vi "Create Read Worker MHLC.vi"(8 "error in (no error)":errorcluster, 10 "Data in":variant, 11 "TCPServer in":refnum<class "DS TCP Server.lvclass">) -> (0 "error out":errorcluster, 3 "TCPServer out":refnum<class "DS TCP Server.lvclass">)   [LabVIEW 2017, in "DS TCP Server.lvlib" / "DS TCP Server.lvclass"]
doc: "Launch a TCP Read Worker to receive incoming data from a Debug Client"
uses:
  DS TCP Server.lvclass
  C:/Program Files (x86)/National Instruments/LabVIEW 2017/vi.lib/addons/_Workers/Library/Classes/Worker/Worker.lvclass
  rql_Create Read Worker.ctl
  <vilib>/addons/_Workers/Library/Classes/Message Queue/Message Queue.lvclass
  Common VIs/DC_UID.ctl
  <vilib>/addons/_Workers/Library/Classes/Message/Priority.ctl
  DS TCP Server.lvclass/DS TCP Server.ctl
  DS TCP Read/Initialization Data.ctl
  DS TCP Read/Response Cases.ctl
  <vilib>/addons/_Workers/Library/Case Label.ctl
  rsp_Connection Notify.ctl
  <vilib>/Utility/error.llb/Error Cluster From Error Code.vi
  <vilib>/ErrorRing/Error Ring.xnode
  DS TCP Read/DS TCP Read.lvclass
  <vilib>/addons/_Workers/Library/Workers.lvlib
  <vilib>/addons/_Workers/Library/Classes/Message/Message.lvclass
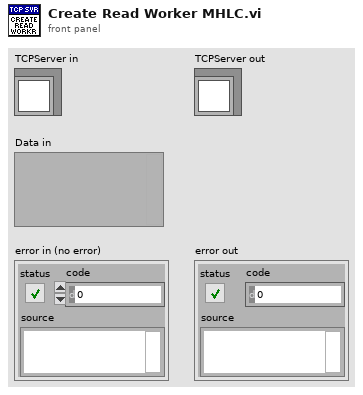
[diagram p1: front panel]
types:
  T1 = typedef "DS TCP Server.lvlib/DS TCP Server.lvclass/rql_Create Read Worker.ctl" = cluster{"Forwarding Q":refnum<class "Message Queue.lvclass">, "DC_UID":T2, "Worker Alias":string, "Message Priority":T3}
  T2 = typedef "DC_UID.ctl" = string
  T3 = typedef "Workers.lvlib/Message.lvclass/Priority.ctl" = enum16{"Low", "Normal", "High"}
  T4 = typedef "DS TCP Server.lvlib/DS TCP Server.lvclass/Connection ID.ctl" = cluster{"Connection Ref":refnum<k5>, "DC_UID":T2, "Message Priority":T3, "IP Address":string}
  T5 = typedef "DS TCP Server.lvlib/DS TCP Server.lvclass/rsp_Connection Notify.ctl" = cluster{"Connected?":bool, "DC_UID":T2, "Message Priority":T3, "IP Address":string}
  T6 = typedef "DS TCP Server.lvlib/DS TCP Read.lvclass/Initialization Data.ctl" = cluster{"Connection ID":refnum<k5>, "Forwarding Queue":refnum<class "Message Queue.lvclass">, "Response Cases":T7}
  T7 = typedef "DS TCP Server.lvlib/DS TCP Read.lvclass/Response Cases.ctl" = cluster{"Connection Lost":T8}
  T8 = typedef "Workers.lvlib/Case Label.ctl" = string
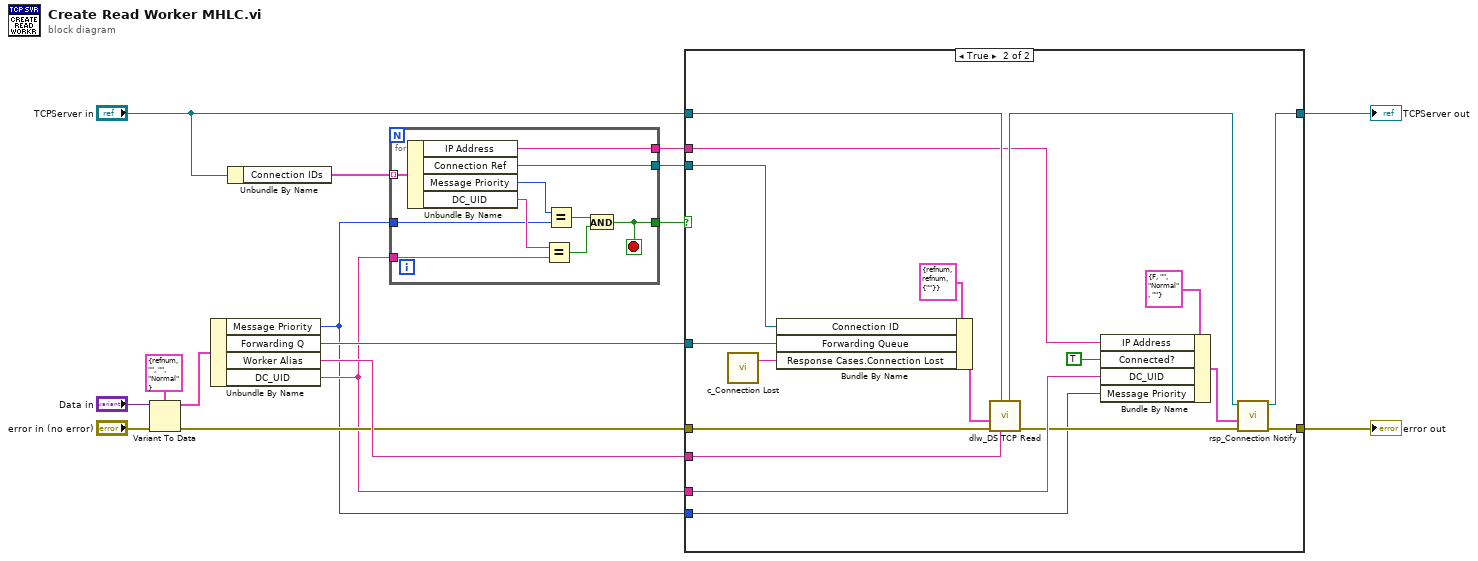
[diagram p0: block diagram]
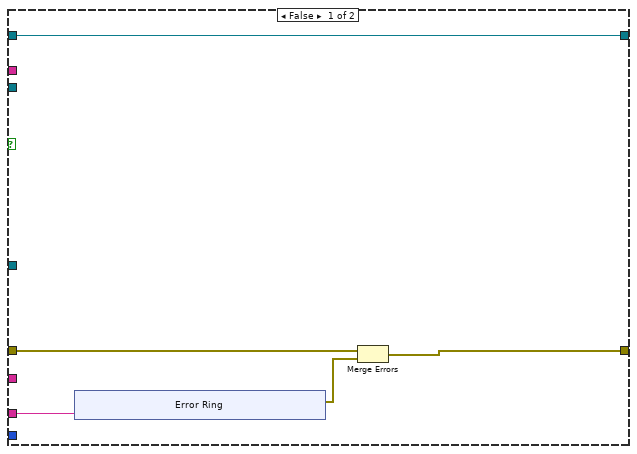
[diagram p2: hidden frame]
diagram:
  n1 = Variant To Data(error in="error in (no error)", type=T1 {"Forwarding Q"=refnum, "DC_UID"="", "Worker Alias"="", "Message Priority"=enum."Normal"} ("Data"), Variant="Data in") -> (data=w10:T1, error out=w7:errorcluster)
  n2 = Unbundle By Name(w10) -> ("Message Priority"=w2:T3, "Forwarding Q"=w11:refnum<class "Message Queue.lvclass">, "Worker Alias"=w12:string, "DC_UID"=w3:T2)
  n3 = Unbundle By Name("TCPServer in") -> ("Connection IDs"=w16:T4[])
  n4 = for {
    tunnel: w16 -> [w26] mode=indexing
    tunnel: w3 -> [w24]
    tunnel: [w18] -> w5
    tunnel: [w23] -> w4
    tunnel: w2 -> [w20]
    tunnel: [w17] -> w1
    stop <- w18 stop-if-true
    n5 = Unbundle By Name(w26) -> ("IP Address"=w17:string, "Connection Ref"=w23:refnum<k5>, "Message Priority"=w21:T3, "DC_UID"=w25:T2)
    n6 = Equal?(x=w25, y=w24) -> (x = y?=w22:bool)
    n7 = Equal?(x=w21, y=w20) -> (x = y?=w19:bool)
    n8 = And(x=w19, y=w22) -> (x .and. y?=w18:bool)
  }
  n9 = case shown="True" w5 {
    tunnel: "TCPServer in" -> [w31 w56]
    tunnel: w3 -> [w28 w55]
    tunnel: [w31 w51] -> w14
    tunnel: [w29 w49] -> w13
    tunnel: w12 -> [_ w48]
    tunnel: w11 -> [_ w46]
    tunnel: w7 -> [w30 w42]
    tunnel: w4 -> [_ w41]
    tunnel: w2 -> [_ w40]
    tunnel: w1 -> [_ w39]
    frame False {
      n10 = xnode "Error Ring"("parameter 0"=w28) -> ("error out"=w27:errorcluster)
      n11 = Merge Errors(w30, w27) -> (w29:errorcluster)
    }
    frame True {
      n12 = call "c_Connection Lost.vi"() -> ("Case Label"=w47:T8)  [unwired: 1 in]
      n13 = Bundle By Name(cluster=T6 {"Connection ID"=refnum, "Forwarding Queue"=refnum, "Response Cases"={"Connection Lost"=""}} ("Initialization Data"), "Connection ID"=w41, "Forwarding Queue"=w46, "Response Cases.Connection Lost"=w47) -> (w45:T6)
      n14 = call "dlw_DS TCP Read.vi"("Worker Alias"=w48, "Caller in"=w56, "error in"=w42, "Initialization Data"=w45) -> ("error out"=w43:errorcluster, "dup Caller out"=w50:refnum<class "DS TCP Server.lvclass">)  [unwired: 5 in, 1 out]
      n15 = Bundle By Name(cluster=T5 {"Connected?"=FALSE, "DC_UID"="", "Message Priority"=enum."Normal", "IP Address"=""} ("Data in"), "IP Address"=w39, "Connected?"=TRUE, "DC_UID"=w55, "Message Priority"=w40) -> (w54:T5)
      n16 = call "rsp_Connection Notify.vi"("error in"=w43, "Data in"=w54, "DS TCP Server in"=w50) -> ("error out"=w49:errorcluster, "dup DS TCP Server out"=w51:refnum<class "DS TCP Server.lvclass">)  [unwired: 7 in]
    }
  }
  "TCPServer out" <- w14
  "error out" <- w13
